vi "UpdateZones.vi"(8 "error in (no error)":errorcluster, 10 "Old Robots":refnum<class "Robot.lvclass">[](array[class]), 11 "object in":refnum<class "Ally.lvclass">) -> (0 "error out":errorcluster, 3 "object out":refnum<class "Ally.lvclass">)   [LabVIEW 2023, in "Ally.lvclass"]
uses:
  Ally.lvclass
  Robot_class/Robot.lvclass
  Ally.lvclass/Ally.ctl
  Robot_class/Robot.lvclass/Robot.ctl
  Robot_class/Read Zone.vi
  Zone_class/Zone.lvclass
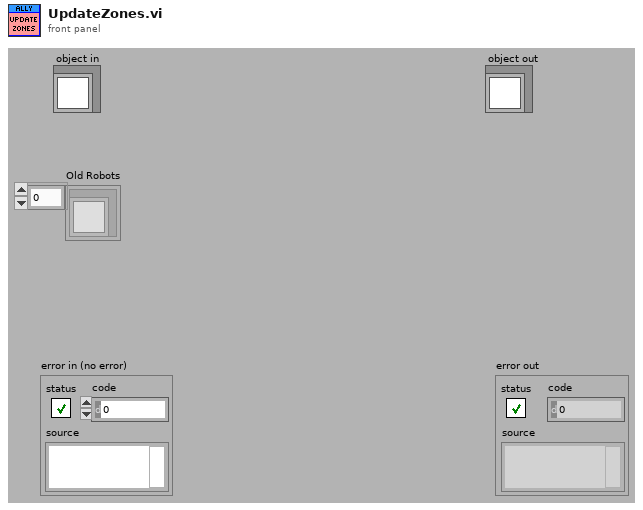
[diagram p1: front panel]
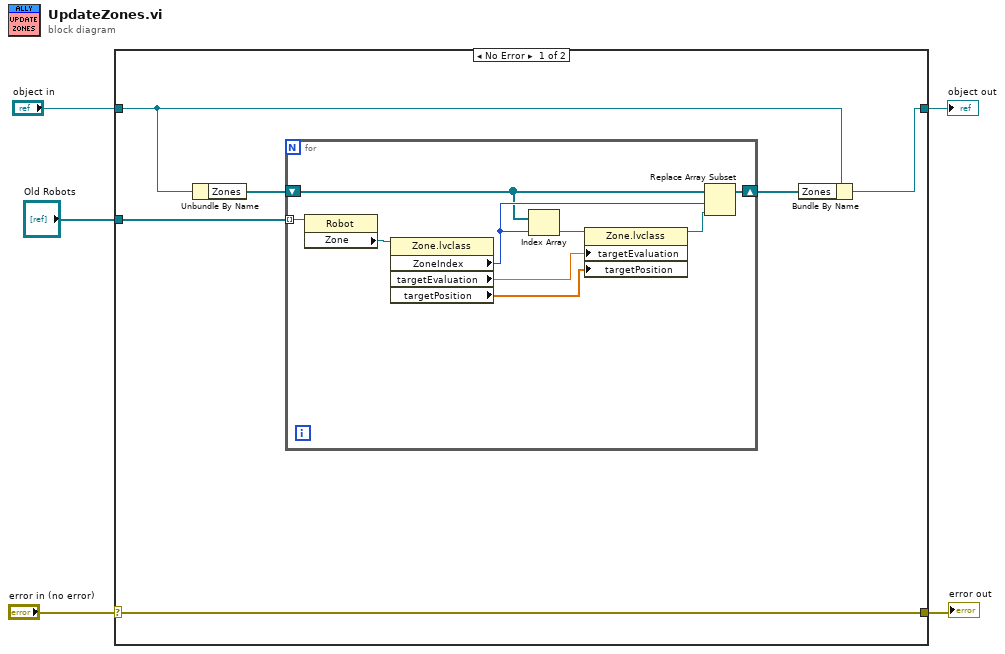
[diagram p0: block diagram]
diagram:
  n1 = case shown="No Error" "error in (no error)" {
    selector: "error in (no error)" -> [w11 w22]
    tunnel: [w11 w22] -> w4
    tunnel: [w7 w21] -> w2
    tunnel: "object in" -> [w8 w21]
    tunnel: "Old Robots" -> [w10 _]
    frame No Error {
      n2 = Unbundle By Name(w8) -> ("Zones"=w9:refnum<class "Zone.lvclass">[])
      n3 = for {
        tunnel: w10 -> [w20] mode=indexing
        shift-right: [w12] -> w6
        shift-left: w9 -> [w17]
        n4 = property class="Robot"(reference=w20) -> ("Zone"=w19:refnum<class "Zone.lvclass">)  [unwired: 1 in, 2 out]
        n5 = property class="Zone.lvclass"(reference=w19) -> ("ZoneIndex"=w18:i32, "targetEvaluation"=w14:dbl, "targetPosition"=w13:dbl[])  [unwired: 1 in, 2 out]
        n6 = Index Array(array=w17, index=w18) -> (element=w15:refnum<class "Zone.lvclass">)
        n7 = property class="Zone.lvclass"(reference=w15, "targetEvaluation"=w14, "targetPosition"=w13) -> (reference out=w16:refnum<class "Zone.lvclass">)  [unwired: 1 in, 1 out]
        n8 = Replace Array Subset(array=w17, new element=w16, index=w18) -> (w12:refnum<class "Zone.lvclass">[])
      }
      n9 = Bundle By Name(cluster=w8, "Zones"=w6) -> (w7:refnum<class "Ally.lvclass">)
    }
    frame Error {
    }
  }
  "error out" <- w4
  "object out" <- w2
